vi "LoopComp.vi"(2 "RandTime":u64 caption="Rand Time (ms)", 3 "LoopPeriod":u64=1 caption="Loop Period (ms)", 4 "SetTime":u64=1000 caption="Set Time (ms)", 5 "LoopCount":u64, 6 "Instance":i32, 7 "Mode":enum16{"Reset", "Run"}(ring)) -> (0 "ActualTime":u64=1000 caption="Actual Time (ms)", 1 "Outcome":enum16{"TimeIn", "TimeOut"}(ring))   [LabVIEW 2013]
panel:
  out "InternalTime":u64[](array[numeric])
  out "RandCount":dbl[](array[numeric])
  out "SetCount":dbl[](array[numeric])
  in  "BaseCount":u64[](array[numeric])=[0, 0, 0, 0, 0, 0, 0, 0, 0, 0]
  # "Internal Variables"
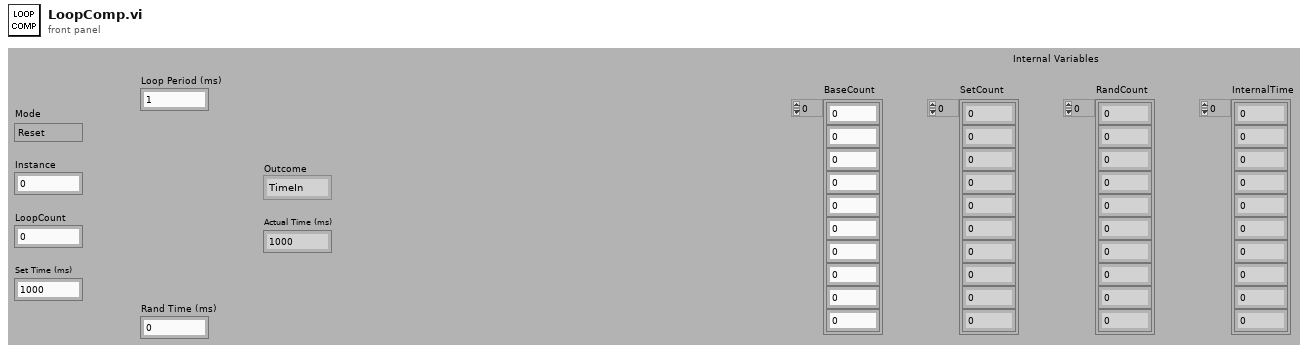
[diagram p1: front panel]
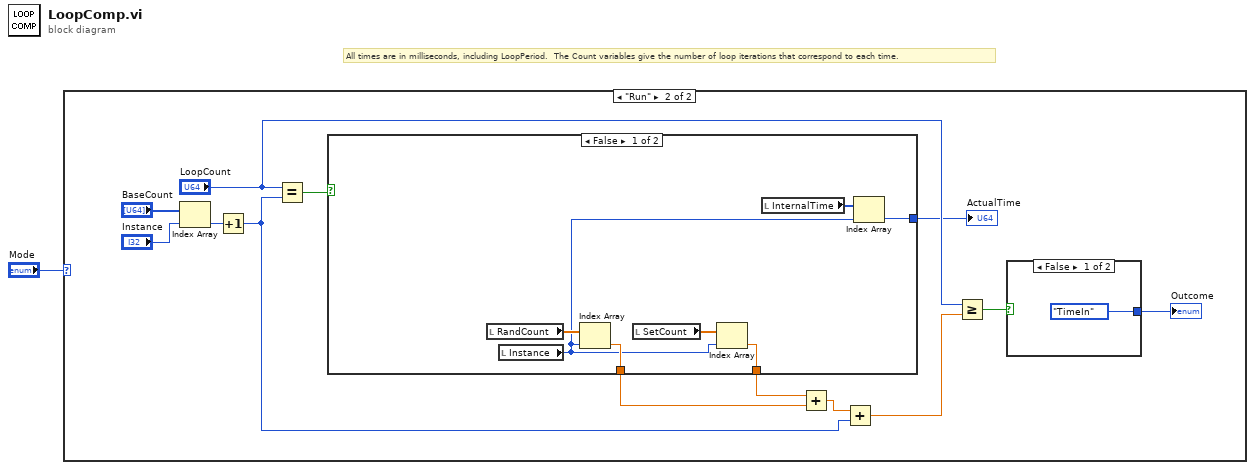
[diagram p0: block diagram]
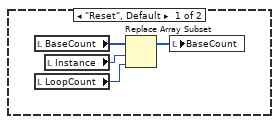
[diagram p2: hidden frame]
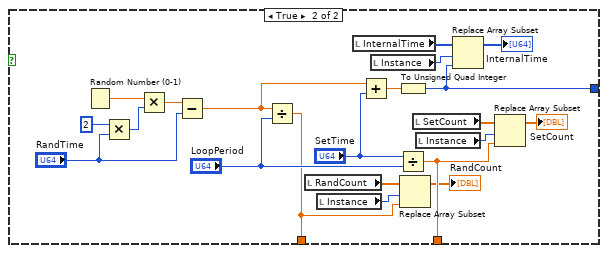
[diagram p3: hidden frame]
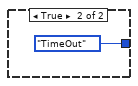
[diagram p4: hidden frame]
diagram:
  # "All times are in milliseconds, including LoopPeriod.  The Count variables give the number of loop iterations that correspond to each time."
  n1 = case shown="\"Run\"" "Mode" {
    frame "Reset", Default {
      n2 = local read "BaseCount"() -> (w4:u64[])
      n3 = local read "LoopCount"() -> (w2:u64)
      n4 = local read "Instance"() -> (w3:i32)
      n5 = Replace Array Subset(array=w4, new element=w2, index=w3) -> (w5:u64[])
      n6 = local write "BaseCount"(w5) -> ()
    }
    frame "Run" {
      n7 = Index Array(array="BaseCount", index="Instance") -> (element=w6:u64)
      n8 = Increment(x=w6) -> (x+1=w10:u64)
      n9 = Equal?(x="LoopCount", y=w10) -> (x = y?=w15:bool)
      n10 = case shown="False" w15 {
        tunnel: [w24 w34] -> w13
        tunnel: [w22 w31] -> w12
        tunnel: [w20 w27] -> w9
        frame False {
          n11 = local read "RandCount"() -> (w23:dbl[])
          n12 = local read "Instance"() -> (w19:i32)
          n13 = Index Array(array=w23, index=w19) -> (element=w22:dbl)
          n14 = local read "SetCount"() -> (w25:dbl[])
          n15 = Index Array(array=w25, index=w19) -> (element=w24:dbl)
          n16 = local read "InternalTime"() -> (w21:u64[])
          n17 = Index Array(array=w21, index=w19) -> (element=w20:u64)
        }
        frame True {
          n18 = Random Number (0-1)() -> (number: 0 to 1=w46:dbl)
          n19 = Multiply(x=u64 2 ("y"), y="RandTime") -> (x*y=w45:u64)
          n20 = Multiply(x=w46, y=w45) -> (x*y=w44:dbl)
          n21 = Subtract(x=w44, y="RandTime") -> (x-y=w39:dbl)
          n22 = Divide(x=w39, y="LoopPeriod") -> (x/y=w31:dbl)
          n23 = local read "RandCount"() -> (w32:dbl[])
          n24 = local read "Instance"() -> (w33:i32)
          n25 = local read "InternalTime"() -> (w28:u64[])
          n26 = Add(x=w39, y="SetTime") -> (x+y=w38:dbl)
          n27 = local read "Instance"() -> (w29:i32)
          n28 = To Unsigned Quad Integer(1:w38) -> (0:w27:u64)
          n29 = Divide(x="SetTime", y="LoopPeriod") -> (x/y=w34:dbl)
          n30 = Replace Array Subset(array=w32, new element=w31, index=w33) -> (→"RandCount":dbl[])
          n31 = local read "SetCount"() -> (w36:dbl[])
          n32 = local read "Instance"() -> (w35:i32)
          n33 = Replace Array Subset(array=w28, new element=w27, index=w29) -> (→"InternalTime":u64[])
          n34 = Replace Array Subset(array=w36, new element=w34, index=w35) -> (→"SetCount":dbl[])
        }
      }
      "ActualTime" <- w9
      n35 = Add(x=w13, y=w12) -> (x+y=w17:dbl)
      n36 = Add(x=w17, y=w10) -> (x+y=w16:dbl)
      n37 = Greater Or Equal?(x="LoopCount", y=w16) -> (x >= y?=w18:bool)
      n38 = case shown="False" w18 {
        tunnel: [enum16{"TimeIn", "TimeOut"}."TimeIn" ("Outcome") enum16{"TimeIn", "TimeOut"}."TimeOut" ("Outcome")] -> w11
        frame False {
        }
        frame True {
        }
      }
      "Outcome" <- w11
    }
  }
